vi "Global_GET_INSTRSTATE.vi"() -> ()   [LabVIEW 2015]
panel:
  in  "Cluster":T1
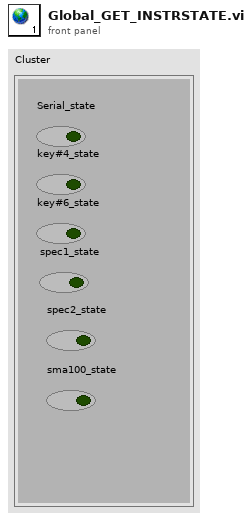
[diagram p1: front panel]
types:
  T1 = cluster{"Serial_state":bool, "key#4_state":bool, "key#6_state":bool, "spec1_state":bool, "spec2_state":bool, "sma100_state":bool}
diagram:
